vi "Open BD.vi"(8 "error in (no error)":errorcluster, 11 "reference":refnum<vi>) -> (0 "error out":errorcluster, 3 "reference out":refnum<vi>)   [LabVIEW 2021]
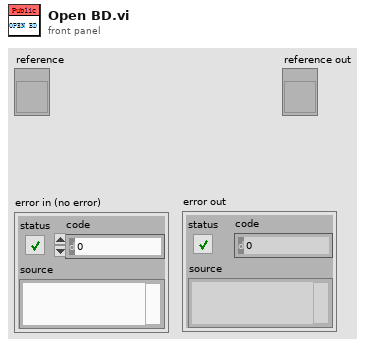
[diagram p1: front panel]
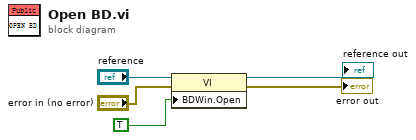
[diagram p0: block diagram]
diagram:
  n1 = property class="VI"(reference="reference", error in="error in (no error)", "BDWin.Open"=TRUE ("Block Diagram Window:Open")) -> (reference out=→"reference out":refnum<vi>, error out=→"error out":errorcluster)
